vi "Actor Core.vi"(8 "error in":errorcluster, 11 "Cooler Panel":refnum<class "Cooler Panel.lvclass">) -> (0 "error out":errorcluster, 3 "Actor out":refnum<class "Actor.lvclass">)   [LabVIEW 2012, in "Cooler UI.lvlib" / "Cooler Panel.lvclass"]
doc: "This is Actor Core.vi, the main message handling loop for Actors. An actor usually just sits in this loop and processes messages as they arrive. Any error returned by the message Do.vi call will stop the loop, with error code 43 as the cannonical signal to stop with no error sent to caller. Descendants may override that in Handle Error.vi."
uses:
  Cooler Panel.lvclass
  <vilib>/ActorFramework/Actor/Actor.lvclass
  Cooler UI with Events/Cooler UI with Events.lvclass/Cooler UI with Events.ctl
  Cooler UI with Events/Cooler UI with Events.lvclass
  <vilib>/ActorFramework/Actor/Actor.lvclass/Actor.ctl
  <vilib>/ActorFramework/Message Enqueuer/Message Enqueuer.lvclass/Message Enqueuer.ctl
  Change Desired Temperature Msg/Change Desired Temperature Msg.lvclass/Change Desired Temperature Msg.ctl
  <vilib>/ActorFramework/Message Enqueuer/Init from Existing Queue.vi
  <vilib>/ActorFramework/Message Enqueuer/Enqueue.vi
  <vilib>/ActorFramework/Message Priority Queue/Priority Enqueue.vi
  <vilib>/ActorFramework/Message Enqueuer/Message Enqueuer.lvclass
  Change Desired Temperature Msg/Change Desired Temperature Msg.lvclass
panel:
  out "Pump":bool
  out "Fault B":bool
  in  "Desired Temperature":dbl=75.0
  out "Temperature":dbl(slide) scale=0.0..120.0
  out "Fault A":bool
  out "Fan B":bool
  out "Fan A":bool
  # "Fan starts 5 seconds after pump starts"
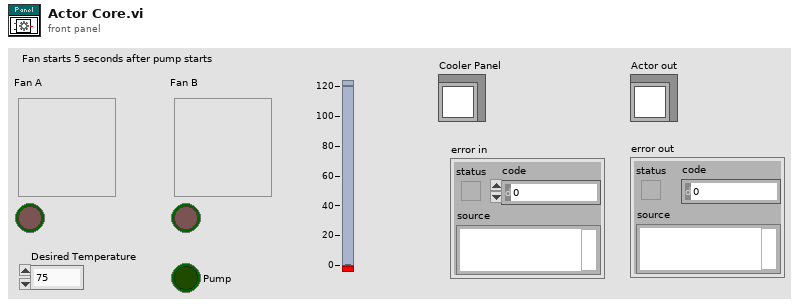
[diagram p1: front panel]
types:
  T1 = enum32{"Invalid", "Standard", "Closed", "Hidden", "Minimized", "Maximized"}
  T2 = typedef "Cooler UI.lvlib/Cooler UI with Events.lvclass/Events.ctl" = cluster{"Fan Status":refnum<user-event>, "Temperature":refnum<user-event>, "Pump":refnum<user-event>}
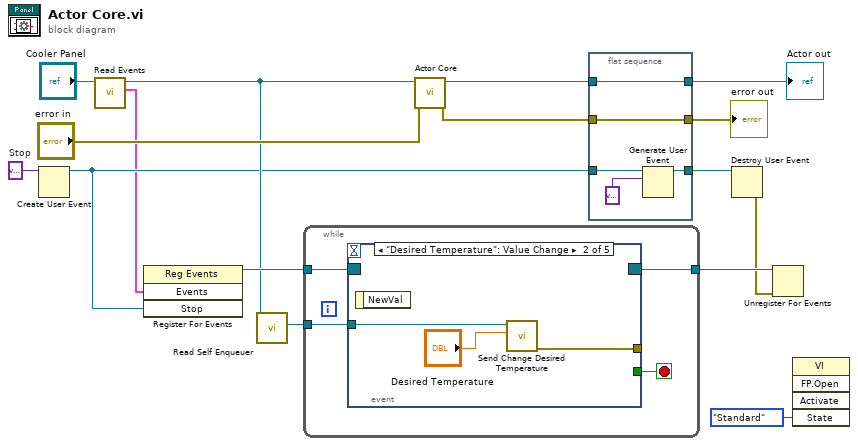
[diagram p0: block diagram]
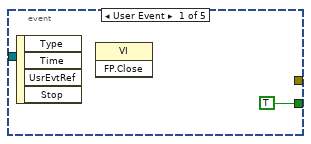
[diagram p2: hidden frame]
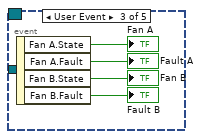
[diagram p3: hidden frame]
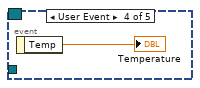
[diagram p4: hidden frame]
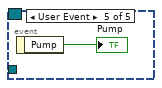
[diagram p5: hidden frame]
diagram:
  w14 = variant  # Stop
  n1 = Create User Event(user event datatype=w14) -> (user event=w3:refnum<user-event>)  [unwired: 1 in, 1 out]
  n2 = call "Read Events.vi"("Cooler UI with Events in"="Cooler Panel") -> ("Events"=w2:T2, "Cooler UI with Events out"=w4:refnum<class "Cooler Panel.lvclass">)  [unwired: 9 in]
  n3 = register-events(w2, w3) -> (reference out=w15:refnum<event-registration>)  [unwired: 2 in, 1 out]
  n4 = call <vilib>:"Read Self Enqueuer.vi"("Actor"=w4) -> ("Self Enqueuer"=w7:refnum<class "Message Enqueuer.lvclass">)  [unwired: 10 in]
  n5 = while {
    tunnel: w15 -> [w20]
    tunnel: [w19] -> w13
    tunnel: w7 -> [w17]
    stop <- w18 stop-if-true
    n6 = event shown="[1] \"Desired Temperature\": Value Change" {
      selector: w20 -> [_ _ _ _ _]
      dyn-events: [_ _ _ _ _] -> w19
      timeout: _ -> [_ _ _ _ _]
      tunnel: [TRUE _ _ _ _] -> w18
      tunnel: w17 -> [_ w24 _ _ _]
      tunnel: [_ w22 _ _ _] -> _
      event User Event {
        n7 = event-data() -> ()  [unwired: 1 in, 4 out]
        n8 = invoke class="VI" method="FP.Close"() -> ()  [unwired: 3 in, 3 out]
      }
      event "Desired Temperature": Value Change {
        n9 = event-data() -> ()  [unwired: 1 in, 1 out]
        n10 = call "Send Change Desired Temperature.vi"("Set Point"="Desired Temperature", "enqueuer"=w24) -> ("error out"=w22:errorcluster)  [unwired: 9 in]
      }
      event User Event {
        n11 = event-data() -> ("Fan A.State"=→"Fan A":bool, "Fan A.Fault"=→"Fault A":bool, "Fan B.State"=→"Fan B":bool, "Fan B.Fault"=→"Fault B":bool)  [unwired: 1 in]
      }
      event User Event {
        n12 = event-data() -> ("Temp"=→"Temperature":dbl)  [unwired: 1 in]
      }
      event User Event {
        n13 = event-data() -> ("Pump"=→"Pump":bool)  [unwired: 1 in]
      }
    }
  }
  n14 = call-parent "Actor Core.vi"("error in"="error in", "Actor in"=w4) -> ("error out"=w1:errorcluster, "Actor out"=w9:refnum<class "Actor.lvclass">)  [unwired: 8 in]
  n15 = flat-sequence {
    tunnel: [w35] -> w11
    tunnel: w3 -> [w34]
    tunnel: w9 -> [w33]
    tunnel: [w33] -> w10
    tunnel: w1 -> [w32]
    tunnel: [w32] -> w8
    frame #0 {
      n16 = Generate User Event(user event=w34, event data cluster=variant ("Stop")) -> (user event out=w35:refnum<user-event>)  [unwired: 1 in, 1 out]
    }
  }
  n17 = Destroy User Event(user event=w11) -> (error out=w12:errorcluster)  [unwired: 1 in]
  n18 = Unregister For Events(event registration refnum=w13, error in=w12) -> ()  [unwired: 1 out]
  n19 = invoke class="VI" method="FP.Open"("State"=T1."Standard") -> ()  [unwired: 4 in, 5 out]
  "error out" <- w8
  "Actor out" <- w10
